vi "test laser.vi"   [LabVIEW 2015]
uses:
  <vilib>/ActorFramework/Actor/Actor.lvclass
  Hardware/Laser Quantum/Laser Quantum.lvclass
  Type Defs/Excitation.ctl
  Type Defs/Laser Configuration.ctl
  Hardware/Laser Quantum Messages/Set Laser Power Msg/Set Laser Power Msg.lvclass
  <vilib>/ActorFramework/Stop Msg/Stop Msg.lvclass
types:
  T1 = typedef "Excitation.ctl" = enum16{"Cy2 (473 nm)", "Cy3 (532 nm)", "Cy5 (639 nm)", "Cy7 (730 nm)"}
  T2 = typedef "Laser Configuration.ctl" = cluster{"Excitation":T1, "Serial Port":refnum<visa-resource-name>}
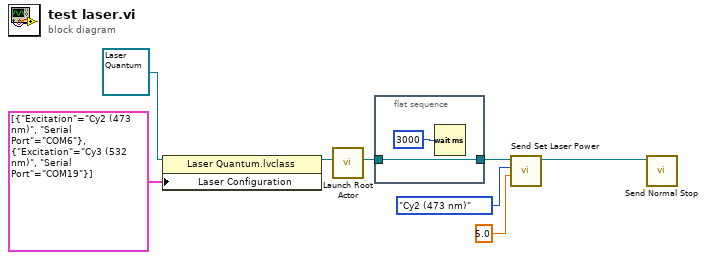
[diagram p0: block diagram]
diagram:
  n1 = property class="Laser Quantum.lvclass"(reference=refnum<class "Laser Quantum.lvclass"> refnum ("Laser Quantum.lvlib:Laser Quantum.lvclass"), "Laser Configuration"=T2[] [{"Excitation"=enum."Cy2 (473 nm)", "Serial Port"="COM6"}, {"Excitation"=enum."Cy3 (532 nm)", "Serial Port"="COM19"}]) -> (reference out=w6:refnum<class "Laser Quantum.lvclass">)  [unwired: 1 in, 1 out]
  n2 = call <vilib>:"Launch Root Actor.vi"("Actor"=w6) -> ("Actor's Enqueuer"=w5:refnum<class "Message Enqueuer.lvclass">)  [unwired: 9 in, 1 out]
  n3 = flat-sequence {
    tunnel: w5 -> [w9]
    tunnel: [w9] -> w4
    frame #0 {
      n4 = Wait (ms)(milliseconds to wait=u32 3000) -> ()  [unwired: 1 out]
    }
  }
  n5 = call "Send Set Laser Power.vi"("Power"=5.0, "Excitation"=Excitation."Cy2 (473 nm)", "Message Enqueuer"=w4) -> ("Message Enqueuer out"=w1:refnum<class "Message Enqueuer.lvclass">)  [unwired: 7 in, 1 out]
  n6 = call <vilib>:"Send Normal Stop.vi"("Message Enqueuer"=w1) -> ()  [unwired: 10 in, 1 out]
